vi "Wheel Type Ring to String.vi"(11 "wheel type_ring":T1 items=["Fixed", "Steering", "Caster", "Mecanum", "Omni", "<Multiple>"]) -> (3 "wheel type":string)   [LabVIEW 2017, in "NI_Robotics_Configure Steering Frame.lvlib" / "User Defined Frame Subpanel.lvlib"]
uses:
  <vilib>/robotics/Dialog/Configure Steering Frame/User Defined Frame Subpanel/User Defined Frame Subpanel.lvlib
  <vilib>/robotics/Dialog/Configure Steering Frame/Wheel Type.ctl
  <vilib>/robotics/Dialog/Configure Steering Frame/NI_Robotics_Configure Steering Frame.lvlib
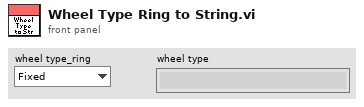
[diagram p1: front panel]
types:
  T1 = typedef "NI_Robotics_Configure Steering Frame.lvlib/Wheel Type.ctl" = u16
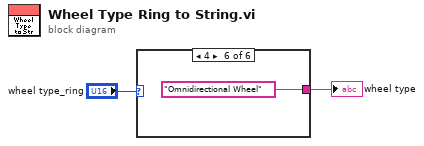
[diagram p0: block diagram]
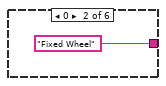
[diagram p3: hidden frame]
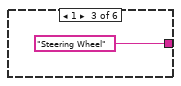
[diagram p4: hidden frame]
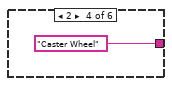
[diagram p5: hidden frame]
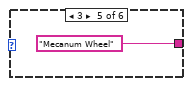
[diagram p6: hidden frame]
diagram:
  n1 = case shown="4" "wheel type_ring" {
    tunnel: [_ "Fixed Wheel" ("wheel type") "Steering Wheel" ("wheel type") "Caster Wheel" ("wheel type") "Mecanum Wheel" ("wheel type") "Omnidirectional Wheel" ("wheel type")] -> w1
    frame Default {
    }
    frame 0 {
    }
    frame 1 {
    }
    frame 2 {
    }
    frame 3 {
    }
    frame 4 {
    }
  }
  "wheel type" <- w1
